vi "STD校准画面.vi"() -> ()   [LabVIEW 2016, in "斯坦道原位多参数.lvlib"]
panel:
  out "B":dbl caption="校准值B:"
  out "K":dbl caption="校准值K:"
  in  "获取温度值":bool
  in  "温度确认校准":bool
  in  "获取温度KB":bool
  in  "拟合计算":bool
  in  "确认校准":bool
  in  "获取KB":bool
  in  "Bt":sgl
  in  "Kt":sgl caption="温度校准参数："
  in  "B值":sgl
  in  "K值":sgl caption="校准参数："
  out "SN":string caption="序列号："
  in  "温度拟合计算":bool
  in  "实际温度":sgl caption="实际温度："
  out "校准记录":string
  in  "第二点取值":bool
  in  "第一点取值":bool
  out "实时信号值":sgl caption="信号值："
  out "实时检测值":sgl caption="检测值："
  in  "第二点信号值":sgl
  in  "第二点标准值":sgl caption="第二点："
  in  "第一点信号值":sgl
  in  "第一点标准值":sgl caption="第一点："
  out "传感器温度":sgl caption="传感器温度："
  in  "校准类型":u16(ring)=2 caption="校准类型：" items=["单点校准"=1, "两点校准"=2]
  in  "校准探头":u16(ring)=10 caption="校准探头：" items=["pH"=10, "溶解氧"=18, "电导率"=12, "浊度"=13, "叶绿素a"=14, "藻密度"=15]
  # "探头校准"
  # "标准值"
  # "信号值"
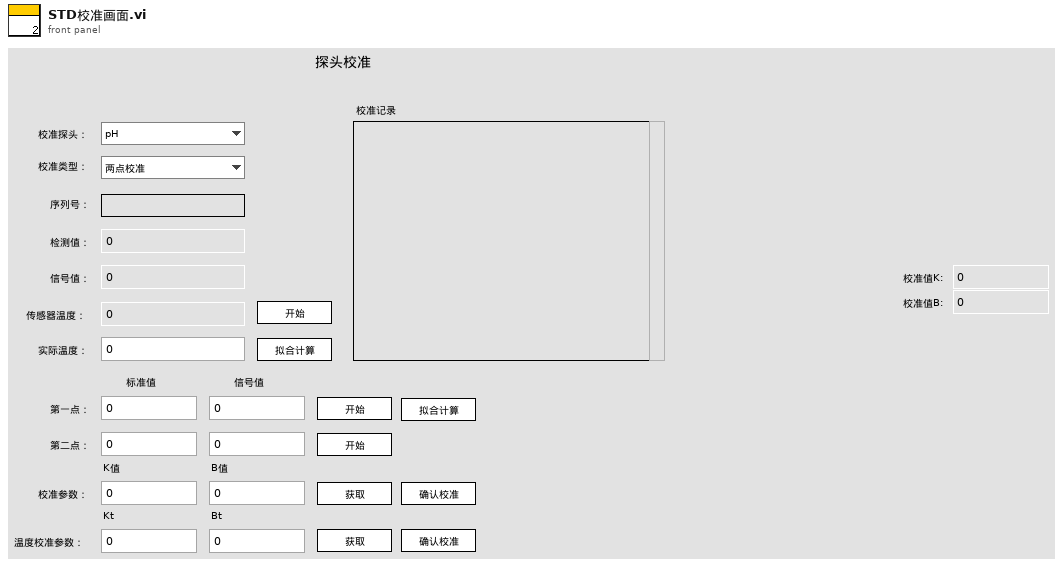
[diagram p1: front panel]
types:
  T1 = cluster{"SN":string, "时间标识":timestamp, "校准类型":u16, "传感器温度":sgl, "第一点标准值":sgl, "第二点标准值":sgl, "第三点标准值":sgl, "第一点检测值":sgl, "第二点检测值":sgl, "第三点检测值":sgl, "第一点原始值":sgl, "第二点原始值":sgl, "第三点原始值":sgl}
  T2 = typedef "校准日志字段定义.ctl" = cluster{"时间":timestamp, "参数":string, "日志信息":string, "流程参数":string}
  T3 = cluster{"SN":string, "时间标识":timestamp, "校准类型":u16, "传感器温度":sgl, "K":sgl, "B":sgl, "Kt":sgl, "Bt":sgl, "第二点检测值":sgl, "第三点检测值":sgl, "第一点原始值":sgl, "第二点原始值":sgl, "第三点原始值":sgl}
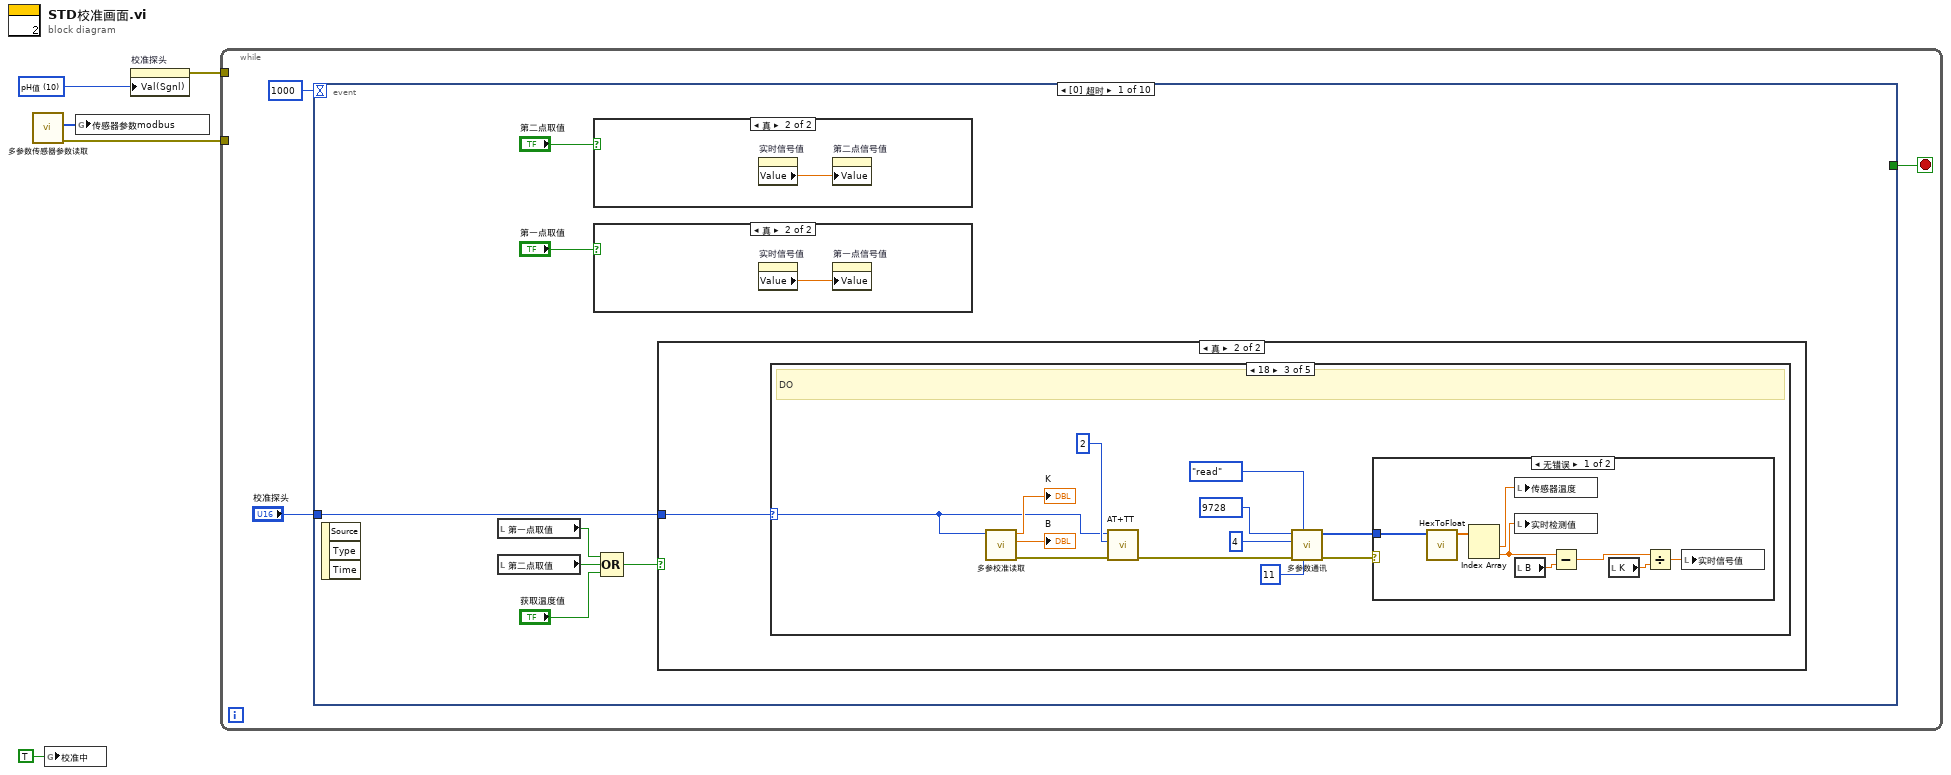
[diagram p0: block diagram]
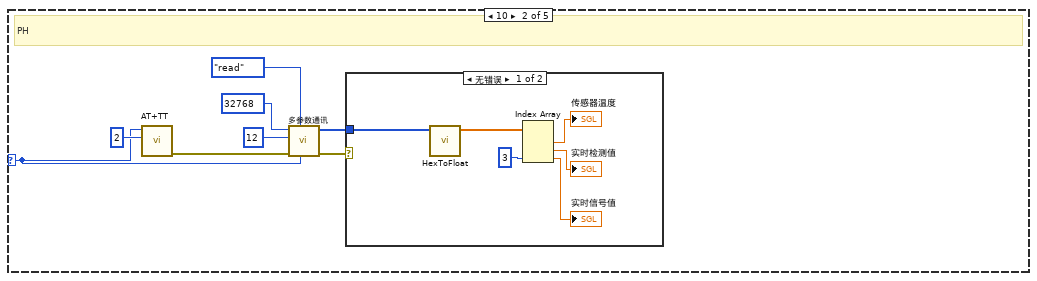
[diagram p4: hidden frame]
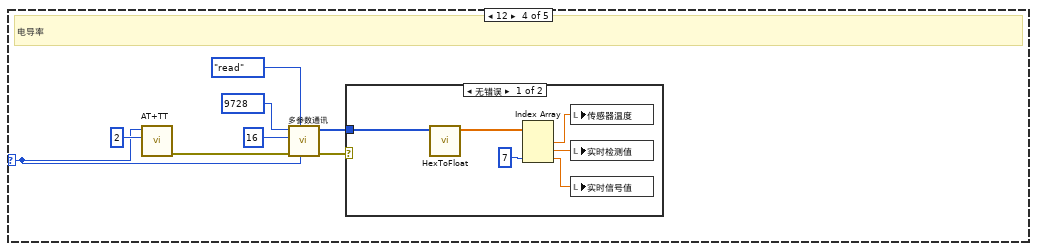
[diagram p7: hidden frame]
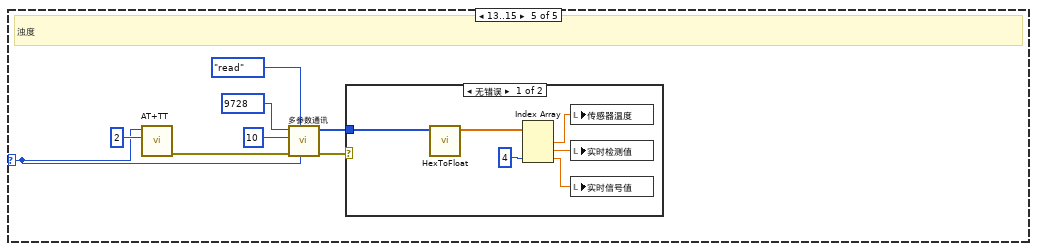
[diagram p9: hidden frame]
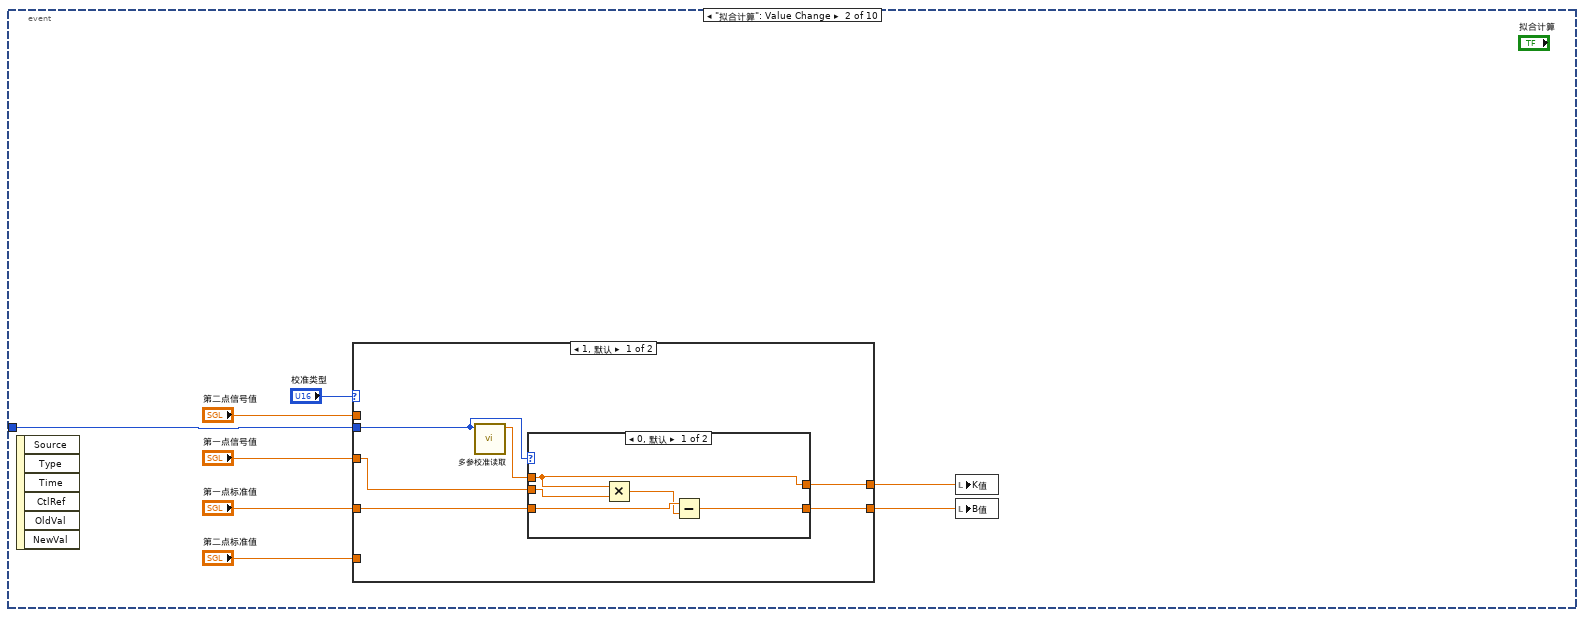
[diagram p13: hidden frame]
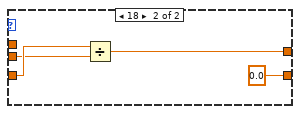
[diagram p14: hidden frame]
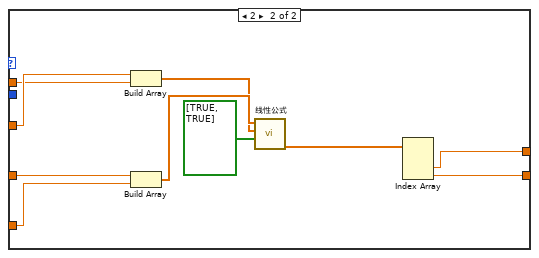
[diagram p15: hidden frame]
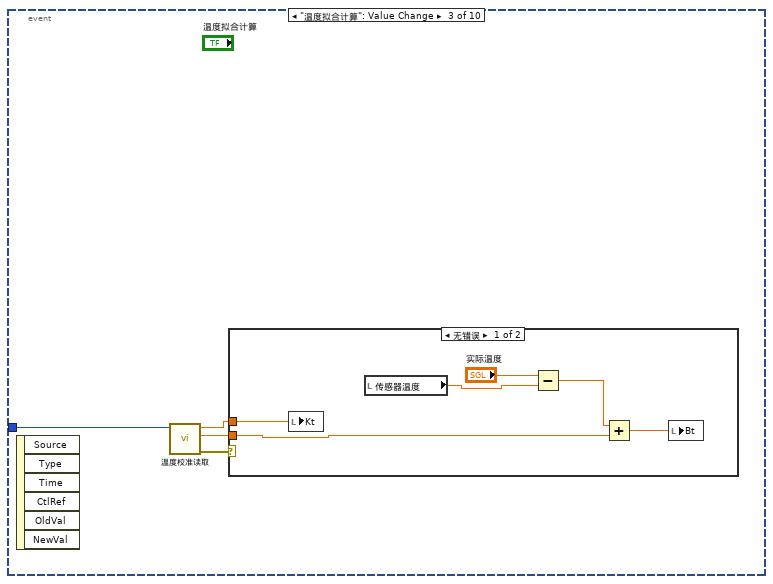
[diagram p16: hidden frame]
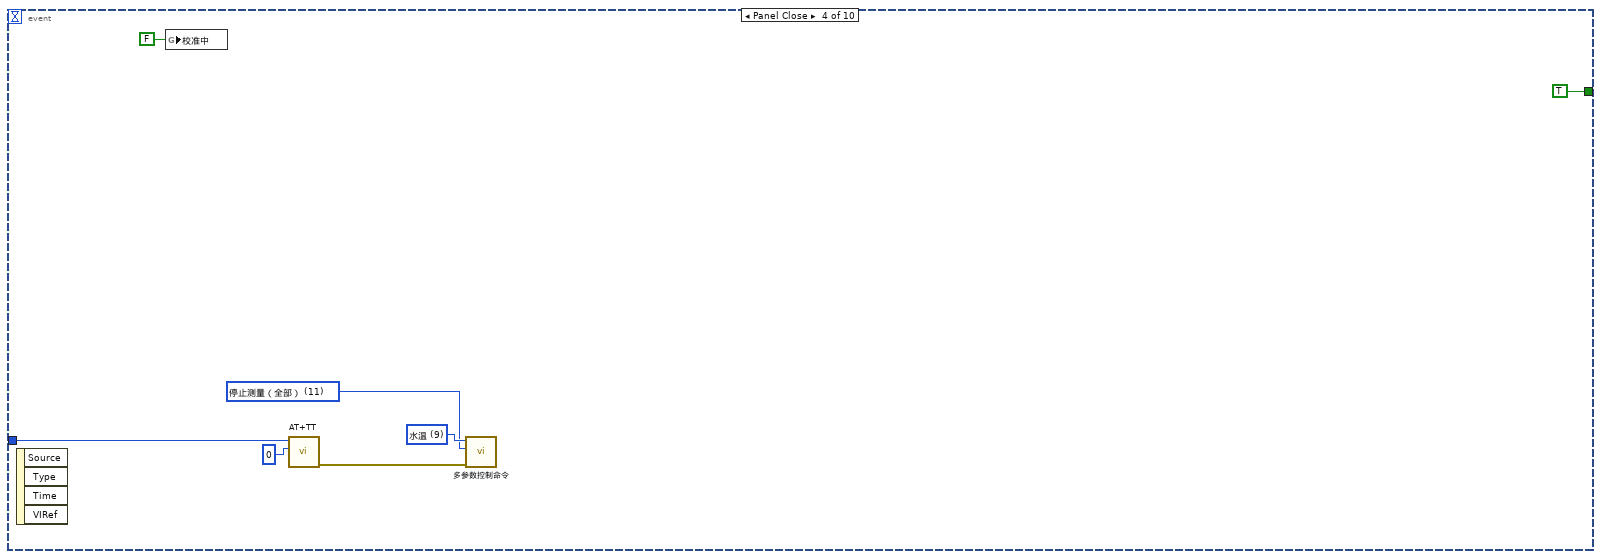
[diagram p18: hidden frame]
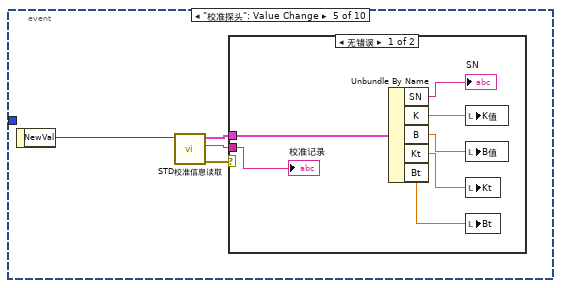
[diagram p19: hidden frame]
diagram:
  w1 = u16 10 items=["pH值"=10, "溶解氧"=18, "电导率"=12, "浊度"=13, "叶绿素a"=14, "藻密度"=15] ("校准探头")
  n1 = call "多参数传感器参数读取.vi"() -> ("error out"=w3:errorcluster, "modbus"=w4:u16[])  [unwired: 9 in, 1 out]
  n2 = global write "多参数全局变量.vi" "校准中"(TRUE ("校准中")) -> ()
  n3 = global write "多参数断电保存全局变量.vi" "传感器参数modbus"(w4) -> ()
  n4 = property on="校准探头" class="Ring (严格)"("Val(Sgnl)"=w1) -> (error out=w2:errorcluster)  [unwired: 2 in, 1 out]
  n5 = while {
    tunnel: w3 -> [_]
    tunnel: w2 -> [_]
    stop <- w8 stop-if-true
    n6 = event shown="[0] 超时" {
      selector: _ -> [_ _ _ _ _ _ _ _ _ _]
      dyn-events: _ -> [_ _ _ _ _ _ _ _ _ _]
      timeout: 1000 -> [_ _ _ _ _ _ _ _ _ _]
      tunnel: [_ _ _ TRUE _ _ _ _ _ _] -> w8
      tunnel: "校准探头" -> [w15 w81 w117 w128 _ _ w150 w159 w167 w191]
      event Timeout {
        n7 = event-data() -> ()  [unwired: 1 in, 3 out]
        n8 = local read "第一点取值"() -> (w11:bool)
        n9 = local read "第二点取值"() -> (w12:bool)
        n10 = case shown="真" "第二点取值" {
          frame False {
          }
          frame True {
            n11 = property on="实时信号值" class="DigNum (严格)"() -> ("Value"=w79:sgl)  [unwired: 2 in, 2 out]
            n12 = property on="第二点信号值" class="DigNum (严格)"("Value"=w79) -> ()  [unwired: 2 in, 2 out]
          }
        }
        n13 = case shown="真" "第一点取值" {
          frame False {
          }
          frame True {
            n14 = property on="实时信号值" class="DigNum (严格)"() -> ("Value"=w80:sgl)  [unwired: 2 in, 2 out]
            n15 = property on="第一点信号值" class="DigNum (严格)"("Value"=w80) -> ()  [unwired: 2 in, 2 out]
          }
        }
        n16 = Compound Arithmetic op=OR ("复合运算")(w11, w12, "获取温度值") -> (w10:bool)
        n17 = case shown="真" w10 {
          tunnel: w15 -> [_ w16]
          frame False {
          }
          frame True {
            n18 = case shown="18" w16 {
              selector: w16 -> [_ w17 w32 w51 w65]
              frame 0, Default {
              }
              frame 10 {
                # "PH"
                n19 = call "AT+TT.vi"("Count"=2, "站号"=w17) -> ("错误输出"=w19:errorcluster)  [unwired: 8 in, 1 out]
                n20 = call "多参数通讯.vi"("Slave ID"=w17, "STEP"=enum16{"open", "read", "write", "close"}."read", "Error in"=w19, "quantity"=u16 12, "starting address"=u16 32768) -> ("error out"=w20:errorcluster, "Registers"=w24:u16[])  [unwired: 4 in, 1 out]
                n21 = case shown="无错误" w20 {
                  tunnel: w24 -> [w29 _]
                  frame No Error {
                    n22 = call "HexToFloat.vi"("数组"=w29) -> ("FLOAT"=w30:sgl[])  [unwired: 10 in]
                    n23 = Index Array(array=w30, index #3=3 ("索引")) -> (element #1=→"传感器温度":sgl, element #2=→"实时检测值":sgl, element #3=→"实时信号值":sgl)  [unwired: 2 in]
                  }
                  frame Error {
                  }
                }
              }
              frame 18 {
                # "DO"
                n24 = call "多参校准读取.vi"("站号"=w32) -> ("error out"=w31:errorcluster, "B"=→"B":dbl, "K"=→"K":dbl)  [unwired: 8 in]
                n25 = call "AT+TT.vi"("错误输入（无错误）"=w31, "Count"=2, "站号"=w32) -> ("错误输出"=w35:errorcluster)  [unwired: 7 in, 1 out]
                n26 = call "多参数通讯.vi"("Slave ID"=u16 11 ("站号"), "STEP"=enum16{"open", "read", "write", "close"}."read", "Error in"=w35, "quantity"=u16 4, "starting address"=u16 9728) -> ("error out"=w38:errorcluster, "Registers"=w42:u16[])  [unwired: 4 in, 1 out]
                n27 = case shown="无错误" w38 {
                  tunnel: w42 -> [w49 _]
                  frame No Error {
                    n28 = call "HexToFloat.vi"("数组"=w49) -> ("FLOAT"=w50:sgl[])  [unwired: 10 in]
                    n29 = Index Array(array=w50) -> (element #1=w48:sgl, element #2=w47:sgl)  [unwired: 2 in]
                    n30 = local write "传感器温度"(w48) -> ()
                    n31 = local write "实时检测值"(w47) -> ()
                    n32 = local read "B"() -> (w46:dbl)
                    n33 = Subtract(x=w47, y=w46) -> (x-y=w45:dbl)
                    n34 = local read "K"() -> (w44:dbl)
                    n35 = Divide(x=w45, y=w44) -> (x/y=w43:dbl)
                    n36 = local write "实时信号值"(w43) -> ()
                  }
                  frame Error {
                  }
                }
              }
              frame 12 {
                # "电导率"
                n37 = call "AT+TT.vi"("Count"=2, "站号"=w51) -> ("错误输出"=w53:errorcluster)  [unwired: 8 in, 1 out]
                n38 = call "多参数通讯.vi"("Slave ID"=w51, "STEP"=enum16{"open", "read", "write", "close"}."read", "Error in"=w53, "quantity"=u16 16, "starting address"=u16 9728) -> ("error out"=w54:errorcluster, "Registers"=w58:u16[])  [unwired: 4 in, 1 out]
                n39 = case shown="无错误" w54 {
                  tunnel: w58 -> [w63 _]
                  frame No Error {
                    n40 = call "HexToFloat.vi"("数组"=w63) -> ("FLOAT"=w64:sgl[])  [unwired: 10 in]
                    n41 = Index Array(array=w64, index #3=7 ("索引")) -> (element #1=w62:sgl, element #2=w61:sgl, element #3=w60:sgl)  [unwired: 2 in]
                    n42 = local write "传感器温度"(w62) -> ()
                    n43 = local write "实时检测值"(w61) -> ()
                    n44 = local write "实时信号值"(w60) -> ()
                  }
                  frame Error {
                  }
                }
              }
              frame 13..15 {
                # "浊度"
                n45 = call "AT+TT.vi"("Count"=2, "站号"=w65) -> ("错误输出"=w67:errorcluster)  [unwired: 8 in, 1 out]
                n46 = call "多参数通讯.vi"("Slave ID"=w65, "STEP"=enum16{"open", "read", "write", "close"}."read", "Error in"=w67, "quantity"=u16 10, "starting address"=u16 9728) -> ("error out"=w68:errorcluster, "Registers"=w72:u16[])  [unwired: 4 in, 1 out]
                n47 = case shown="无错误" w68 {
                  tunnel: w72 -> [w77 _]
                  frame No Error {
                    n48 = call "HexToFloat.vi"("数组"=w77) -> ("FLOAT"=w78:sgl[])  [unwired: 10 in]
                    n49 = Index Array(array=w78, index #3=4 ("索引")) -> (element #1=w76:sgl, element #2=w75:sgl, element #3=w74:sgl)  [unwired: 2 in]
                    n50 = local write "传感器温度"(w76) -> ()
                    n51 = local write "实时检测值"(w75) -> ()
                    n52 = local write "实时信号值"(w74) -> ()
                  }
                  frame Error {
                  }
                }
              }
            }
          }
        }
      }
      event "拟合计算": Value Change {
        n53 = event-data() -> ()  [unwired: 1 in, 6 out]
        n54 = case shown="1, 默认" "校准类型" {
          tunnel: "第一点标准值" -> [w93 w113]
          tunnel: "第一点信号值" -> [w92 w111]
          tunnel: "第二点标准值" -> [_ w112]
          tunnel: "第二点信号值" -> [_ w110]
          tunnel: [w91 w105] -> w88
          tunnel: [w90 w104] -> w87
          tunnel: w81 -> [w94 _]
          frame 1, Default {
            n55 = call "多参校准读取.vi"("站号"=w94) -> ("K"=w89:dbl)  [unwired: 8 in, 2 out]
            n56 = case shown="0, 默认" w94 {
              tunnel: w93 -> [w99 w103]
              tunnel: w92 -> [w98 w102]
              tunnel: [w97 w101] -> w91
              tunnel: [w95 0.0] -> w90
              tunnel: w89 -> [w97 _]
              frame 0, Default {
                n57 = Multiply(x=w97, y=w98) -> (x*y=w96:dbl)
                n58 = Subtract(x=w99, y=w96) -> (x-y=w95:dbl)
              }
              frame 18 {
                n59 = Divide(x=w103, y=w102) -> (x/y=w101:sgl)
              }
            }
          }
          frame 2 {
            n60 = Build Array(w111, w110) -> (w107:sgl[])
            n61 = Build Array(w113, w112) -> (w108:sgl[])
            n62 = call "线性公式.vi"("启用"=bool[] [TRUE, TRUE], "信号值"=w107, "标液浓度"=w108) -> ("Polynomial Coefficients"=w106:dbl[])  [unwired: 5 in, 3 out]
            n63 = Index Array(array=w106) -> (element #2=w105:dbl, element #3=w104:dbl)  [unwired: 3 in, 1 out]
          }
        }
        n64 = local write "K值"(w88) -> ()
        n65 = local write "B值"(w87) -> ()
      }
      event "温度拟合计算": Value Change {
        n66 = event-data() -> ()  [unwired: 1 in, 6 out]
        n67 = call "温度校准读取.vi"("站号"=w117) -> ("error out"=w114:errorcluster, "Bt"=w115:sgl, "Kt"=w116:sgl)  [unwired: 8 in]
        n68 = case shown="无错误" w114 {
          tunnel: w116 -> [w122 _]
          tunnel: w115 -> [w119 _]
          frame No Error {
            n69 = local write "Kt"(w122) -> ()
            n70 = local read "传感器温度"() -> (w121:sgl)
            n71 = Subtract(x="实际温度", y=w121) -> (x-y=w120:sgl)
            n72 = Add(x=w120, y=w119) -> (x+y=w118:sgl)
            n73 = local write "Bt"(w118) -> ()
          }
          frame Error {
          }
        }
      }
      event Panel Close {
        w124 = u16 11 items=["启动测量（全部）"=1, "初始化（清洗）"=10, "停止测量（全部）"=11, "校时"=13, "启动测量（单个传感器）"=19, "停止测量（单个传感器）"=20] ("控制命令")
        w125 = u16 9 items=["氨氮"=3, "水温"=9, "pH值"=10, "溶解氧"=11, "电导率"=12, "浊度"=13, "叶绿素a"=14, "藻密度"=15, "蓝绿藻"=16, "氧化还原电位"=17, "溶解氧%"=18, "盐度"=19] ("站号")
        n74 = event-data() -> ()  [unwired: 1 in, 4 out]
        n75 = global write "多参数全局变量.vi" "校准中"(FALSE ("校准中")) -> ()
        n76 = call "AT+TT.vi"("Count"=0, "站号"=w128) -> ("错误输出"=w126:errorcluster)  [unwired: 8 in, 1 out]
        n77 = call "多参数控制命令.vi"("Error in"=w126, "控制命令"=w124, "站号"=w125) -> ()  [unwired: 8 in, 1 out]
      }
      event "校准探头": Value Change {
        n78 = event-data() -> ("NewVal"=w132:u16)  [unwired: 1 in]
        n79 = call "STD校准信息读取.vi"("Slave ID"=w132) -> ("error out"=w133:errorcluster, "结果字符串"=w134:string, "校准信息读取"=w131:T3)  [unwired: 8 in]
        n80 = case shown="无错误" w133 {
          tunnel: w134 -> [w141 _]
          tunnel: w131 -> [w135 _]
          frame No Error {
            n81 = Unbundle By Name(w135) -> ("SN"=→"SN":string, "K"=w137:sgl, "B"=w138:sgl, "Kt"=w139:sgl, "Bt"=w140:sgl)
            n82 = local write "K值"(w137) -> ()
            n83 = local write "B值"(w138) -> ()
            n84 = local write "Kt"(w139) -> ()
            n85 = local write "Bt"(w140) -> ()
            "校准记录" <- w141
          }
          frame Error {
          }
        }
      }
      event "第一点标准值", "第一点信号值", "第二点标准值", "第二点信号值", "实际温度", "K值", "B值", "Kt", "Bt": Mouse Down {
        n86 = event-data() -> ("CtlRef"=w145:refnum<vi>)  [unwired: 1 in]
        n87 = property class="DigNum (严格)"(reference=w145) -> (reference out=w142:refnum<vi>, "Value"=w144:sgl)  [unwired: 1 in, 1 out]
        n88 = call "数字键盘.vi"("OldNumber"=w144) -> ("NewNumber"=w143:dbl)
        n89 = property class="DigNum (严格)"(reference=w142, "Value"=w143) -> ()  [unwired: 1 in, 2 out]
      }
      event "获取KB": Value Change {
        n90 = event-data() -> ()  [unwired: 1 in, 6 out]
        n91 = call "多参校准读取.vi"("站号"=w150) -> ("error out"=w148:errorcluster, "B"=w146:dbl, "K"=w147:dbl)  [unwired: 8 in]
        n92 = case shown="无错误" w148 {
          tunnel: ["读取参数成功！" "读取参数失败！"] -> w149
          tunnel: w147 -> [w152 _]
          tunnel: w146 -> [w151 _]
          frame No Error {
            n93 = local write "K值"(w152) -> ()
            n94 = local write "B值"(w151) -> ()
          }
          frame Error {
          }
        }
        n95 = One Button Dialog(message=w149) -> ()  [unwired: 1 in, 1 out]
      }
      event "获取温度KB": Value Change {
        n96 = event-data() -> ()  [unwired: 1 in, 1 out]
        n97 = call "温度校准读取.vi"("站号"=w159) -> ("error out"=w157:errorcluster, "Bt"=w155:sgl, "Kt"=w156:sgl)  [unwired: 8 in]
        n98 = case shown="无错误" w157 {
          tunnel: ["读取参数成功！" "读取参数失败！"] -> w158
          tunnel: w156 -> [w161 _]
          tunnel: w155 -> [w160 _]
          frame No Error {
            n99 = local write "Kt"(w161) -> ()
            n100 = local write "Bt"(w160) -> ()
          }
          frame Error {
          }
        }
        n101 = One Button Dialog(message=w158) -> ()  [unwired: 1 in, 1 out]
      }
      event "温度确认校准": Value Change {
        n102 = event-data() -> ()  [unwired: 1 in, 6 out]
        n103 = local read "传感器温度"() -> (w172:sgl)
        n104 = local read "校准类型"() -> (w174:u16)
        n105 = local read "K值"() -> (w171:sgl)
        n106 = local read "B值"() -> (w170:sgl)
        n107 = local read "SN"() -> (w176:string)
        n108 = Get Date/Time In Seconds() -> (seconds since 1Jan1904=w173:timestamp)
        n109 = local read "Kt"() -> (w169:sgl)
        n110 = local read "Bt"() -> (w168:sgl)
        n111 = Bundle By Name(cluster=T1 {"SN"="", "时间标识"=timestamp(0 s since 1904-01-01), "校准类型"=0, "传感器温度"=0.0, "第一点标准值"=0.0, "第二点标准值"=0.0, "第三点标准值"=0.0, "第一点检测值"=0.0, "第二点检测值"=0.0, "第三点检测值"=0.0, "第一点原始值"=0.0, "第二点原始值"=0.0, "第三点原始值"=0.0} ("校准信息读取"), "SN"=w176, "时间标识"=w173, "校准类型"=w174, "传感器温度"=w172, "第一点标准值"=w171, "第二点标准值"=w170, "第三点标准值"=w169, "第一点检测值"=w168) -> (w175:T1)
        n112 = call "温度校准写入.vi"("B 2"="Bt", "K 2"="Kt", "站号"=w167) -> ("error out"=w166:errorcluster)  [unwired: 8 in]
        n113 = call "STD校准信息写入.vi"("Error in"=w166, "校准信息读取"=w175, "Slave ID"=w167) -> ("error out"=w165:errorcluster, "结果字符串"=w164:string)  [unwired: 7 in]
        n114 = case shown="无错误" w165 {
          tunnel: ["校准写入成功！" "校准写入失败！"] -> w180
          tunnel: w164 -> [w181 _]
          frame No Error {
            (unwired) "校准写入成功！"
            n115 = property on="校准探头" class="Ring (严格)"() -> ("RingText.Text"=w182:string)  [unwired: 2 in, 2 out]
            n116 = Get Date/Time In Seconds() -> (seconds since 1Jan1904=w183:timestamp)
            n117 = Bundle By Name(cluster=T2 {"时间"=timestamp(0 s since 1904-01-01), "参数"="", "日志信息"="", "流程参数"=""} ("data"), "时间"=w183, "参数"=w182, "日志信息"=w181) -> (w184:T2)
            n118 = call "校准日志数据插入.vi"("data"=w184) -> ()  [unwired: 9 in, 1 out]
          }
          frame Error {
          }
        }
        n119 = One Button Dialog(message=w180) -> ()  [unwired: 1 in, 1 out]
      }
      event "确认校准": Value Change {
        n120 = event-data() -> ()  [unwired: 1 in, 6 out]
        n121 = local read "传感器温度"() -> (w196:sgl)
        n122 = local read "校准类型"() -> (w198:u16)
        n123 = local read "K值"() -> (w195:sgl)
        n124 = local read "B值"() -> (w194:sgl)
        n125 = local read "SN"() -> (w200:string)
        n126 = Get Date/Time In Seconds() -> (seconds since 1Jan1904=w197:timestamp)
        n127 = local read "Kt"() -> (w193:sgl)
        n128 = local read "Bt"() -> (w192:sgl)
        n129 = Bundle By Name(cluster=T1 {"SN"="", "时间标识"=timestamp(0 s since 1904-01-01), "校准类型"=0, "传感器温度"=0.0, "第一点标准值"=0.0, "第二点标准值"=0.0, "第三点标准值"=0.0, "第一点检测值"=0.0, "第二点检测值"=0.0, "第三点检测值"=0.0, "第一点原始值"=0.0, "第二点原始值"=0.0, "第三点原始值"=0.0} ("校准信息读取"), "SN"=w200, "时间标识"=w197, "校准类型"=w198, "传感器温度"=w196, "第一点标准值"=w195, "第二点标准值"=w194, "第三点标准值"=w193, "第一点检测值"=w192) -> (w199:T1)
        n130 = call "多参数校准写入.vi"("B"="B值", "K"="K值", "站号"=w191) -> ("error out"=w189:errorcluster)  [unwired: 8 in]
        n131 = call "STD校准信息写入.vi"("Error in"=w189, "校准信息读取"=w199, "Slave ID"=w191) -> ("error out"=w190:errorcluster, "结果字符串"=w188:string)  [unwired: 7 in]
        n132 = case shown="无错误" w190 {
          tunnel: ["校准写入成功！" "校准写入失败！"] -> w204
          tunnel: w188 -> [w205 _]
          frame No Error {
            n133 = property on="校准探头" class="Ring (严格)"() -> ("RingText.Text"=w206:string)  [unwired: 2 in, 2 out]
            n134 = Get Date/Time In Seconds() -> (seconds since 1Jan1904=w207:timestamp)
            n135 = Bundle By Name(cluster=T2 {"时间"=timestamp(0 s since 1904-01-01), "参数"="", "日志信息"="", "流程参数"=""} ("data"), "时间"=w207, "参数"=w206, "日志信息"=w205) -> (w208:T2)
            n136 = call "校准日志数据插入.vi"("data"=w208) -> ()  [unwired: 9 in, 1 out]
          }
          frame Error {
          }
        }
        n137 = One Button Dialog(message=w204) -> ()  [unwired: 1 in, 1 out]
      }
    }
  }
